vi "Set Instrument Status.vi"(8 "error in (no error)":errorcluster, 9 "Value (0)":u8, 10 "Instrument Status (0: Standard Event Status Enable Register)":u16(ring) items=["Standard Event Status Enable Register", "Service Request Enable Register", "Operation Complete Bit", "Wait"], 11 "VISA resource name":refnum<visa-resource-name>) -> (0 "error out":errorcluster, 3 "VISA resource name out":refnum<visa-resource-name>)   [LabVIEW 2017, in "HH PLI Series.lvlib"]
doc: "Sets different instrument status register.\n\n<b>Note</b>\nRefer to manual for details about the status register system."
uses:
  HH PLI Series.lvlib
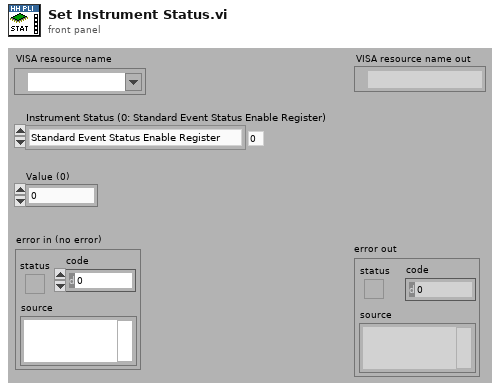
[diagram p1: front panel]
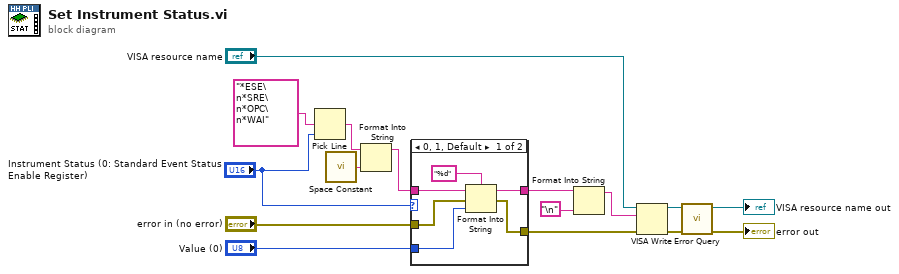
[diagram p0: block diagram]
diagram:
  n1 = Pick Line(multi-line string="*ESE\n*SRE\n*OPC\n*WAI", line index="Instrument Status (0: Standard Event Status Enable Register)") -> (output string=w4:string)  [unwired: 1 in]
  n2 = call <vilib>:"Space Constant.vi"() -> ("String"=w5:string)
  n3 = Format Into String(initial string=w4, w5) -> (resulting string=w6:string)  [unwired: 2 in, 1 out]
  n4 = case shown="0, 1, Default" "Instrument Status (0: Standard Event Status Enable Register)" {
    tunnel: "Value (0)" -> [w22 _]
    tunnel: "error in (no error)" -> [w21 w23]
    tunnel: [w20 w23] -> w13
    tunnel: [w19 w24] -> w2
    tunnel: w6 -> [w18 w24]
    frame 0, 1, Default {
      n5 = Format Into String(format string="%d", initial string=w18, error in=w21, w22) -> (resulting string=w19:string, error out=w20:errorcluster)
    }
    frame 2, 3 {
    }
  }
  n6 = Format Into String(initial string=w2, "\n") -> (resulting string=w1:string)  [unwired: 2 in, 1 out]
  n7 = VISA Write(VISA resource name="VISA resource name", write buffer=w1, error in (no error)=w13) -> (VISA resource name out=w12:refnum<visa-resource-name>, error out=w11:errorcluster)  [unwired: 1 out]
  n8 = call "Error Query.vi"("error in (no error)"=w11, "VISA resource name"=w12) -> ("error out"=→"error out":errorcluster, "VISA resource name out"=→"VISA resource name out":refnum<visa-resource-name>)  [unwired: 6 in, 2 out]
